vi "TestSin.vi"() -> ()   [LabVIEW 2016]
uses:
  controls/Enum.ctl
  <vilib>/Utility/error.llb/Error Cluster From Error Code.vi
  <vilib>/rvi/errors/niLvFpgaAdjustHostInterfaceError.vi
  <vilib>/rvi/interface/nirviReadWriteControl/nirviReadWriteControl.xnode
  controls/FPGAVIreferenceTypeDef.ctl
  FPGA Bitfiles/qnmController797_usbRIO_controllerFPGAmu.lvbitx
  <vilib>/measure/NI_MABase.lvlib
  NiFpgaLv.dll
panel:
  in  "sampling info":cluster{"Fs":dbl, "#s":dbl}={"Fs"=1000.0, "#s"=1000.0} {"Fs" format="%.2p"}
  in  "stop":bool
  out "Waveform Chart":dbl(graph)
  in  "amplitude":dbl=1.0 format="%0.2p"
  in  "frequency":dbl=10.0 format="%0.2p"
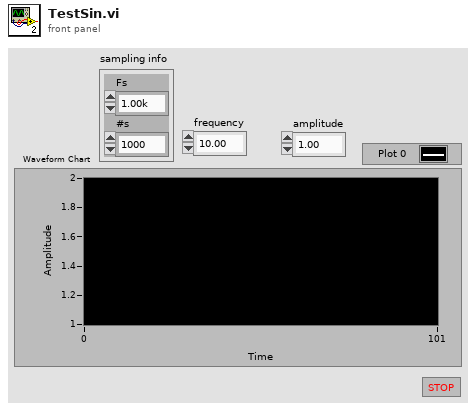
[diagram p1: front panel]
types:
  T1 = typedef "Enum.ctl" = enum16{"Init", "Read", "Write"}
  T2 = typedef "FPGAVIreferenceTypeDef.ctl" = refnum<k20>
  T3 = enum16{"Sine Wave", "Triangle Wave", "Square Wave", "Sawtooth Wave"}
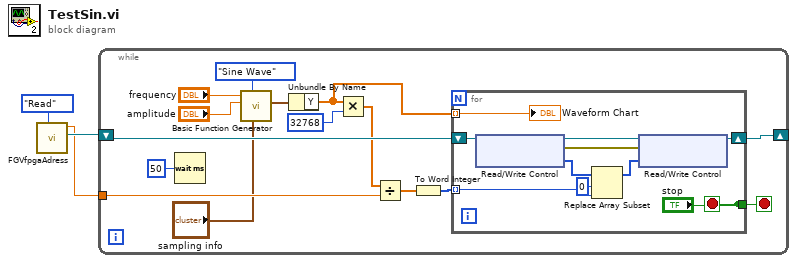
[diagram p0: block diagram]
diagram:
  n1 = call "FGVfpgaAdress.vi"("Enum"=Enum."Read") -> ("FPGA VI Reference Out"=w2:T2, "voltageRange(+/-)Out"=w1:dbl)  [unwired: 6 in, 3 out]
  n2 = while {
    tunnel: w1 -> [w17]
    shift-right: [w16] -> _
    shift-left: w2 -> [w15]
    stop <- w5 stop-if-true
    n3 = Wait (ms)(milliseconds to wait=u32 50) -> ()  [unwired: 1 out]
    n4 = call <vilib>:"Basic Function Generator.vi"("sampling info"="sampling info", "signal type"=T3."Sine Wave", "amplitude"="amplitude", "frequency"="frequency") -> ("signal out"=w11:waveform(dbl))  [unwired: 5 in, 2 out]
    n5 = Unbundle By Name(w11) -> ("Y"=w6:dbl[])
    n6 = Multiply(x=w6, y=32768) -> (x*y=w10:dbl[])
    n7 = Divide(x=w10, y=w17) -> (x/y=w8:dbl[])
    n8 = To Word Integer(number=w8) -> (16bit integer=w7:i16[])
    n9 = for {
      shift-right: [w28] -> w16
      shift-left: w15 -> [w27]
      tunnel: w7 -> [w22] mode=indexing
      tunnel: w6 -> [w20] mode=indexing
      tunnel: ["stop"] -> w5
      stop <- "stop" stop-if-true
      n10 = xnode "Read/Write Control"("FPGA VI Reference In"=w27) -> ("FPGA VI Reference Out"=w26:T2, "error out"=w25:errorcluster, "aio.o.outputs"=w24:i16[])  [unwired: 1 in]
      n11 = Replace Array Subset(array=w24, new element=w22, index=0) -> (w23:i16[])
      n12 = xnode "Read/Write Control"("FPGA VI Reference In"=w26, "error in"=w25, "aio.o.outputs"=w23) -> ("FPGA VI Reference Out"=w28:T2)  [unwired: 1 out]
      "Waveform Chart" <- w20
    }
  }
